vi "Z6_Beamline.color Beamline.vi"(0 "i ref in":refnum<vi>, 5 "error in (no error)":errorcluster) -> (14 "i ref out":refnum<vi>, 19 "error out":errorcluster)   [LabVIEW 2014, in "Z6_Beamline.lvlib"]
doc: "This VI sets the color of several beamline elements."
uses:
  Z6_Beamline.lvlib
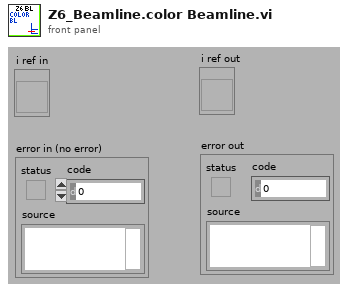
[diagram p1: front panel]
types:
  T1 = typedef "Z6_Beamline.lvlib/Z6_Beamline.i attribute.ctl" = cluster{"Subs ok GUI Refs":T2, "Refs BL Northtower":refnum<vi>[], "Refs BL Southtower":refnum<vi>[], "Refs BL 100TW COS":refnum<vi>[], "State Subsystems":cluster{"Northtower":bool, "Southtower":bool, "Frontends":bool, "100TW COS":bool}, "Z6 Beamline Status Subscriber Information":T3, "Color State PHELIX":i16}
  T2 = typedef "Z6_Beamline.lvlib/Z6_Beamline.Subsystem ok GUI Refs.ctl" = cluster{"Northtower ok":refnum<vi>, "Southtower ok":refnum<vi>, "Frontends ok":refnum<vi>, "100TW COS ok":refnum<vi>}
  T3 = typedef "Z6_Beamline.lvlib/Z6_Beamline.Status Subscriber Information.ctl" = cluster{"BL Z6 Shutter":T4, "CH 10":T4, "CH 11":T4, "ST Flip Cam":T4, "ST Flip DB":T4, "BL Z6 Dump":T4}
  T4 = typedef "PH_BL-Master.lvlib/PH_BL-Master.Status Subscriber Information.ctl" = cluster{"Index of element":i32, "Attributeset":T5}
  T5 = typedef "PH_BL-Master.lvlib/PH_BL-Master.Attribute Set.ctl" = enum16{"Boolean Status Service Subscriber", "Picture Status Service Subscriber"}
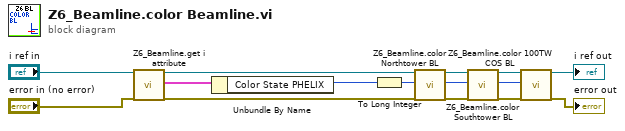
[diagram p0: block diagram]
diagram:
  n1 = call "Z6_Beamline.get i attribute.vi"("i ref in"="i ref in", "error in (no error)"="error in (no error)") -> ("i ref out"=w10:refnum<vi>, "i attribute"=w7:T1, "error out"=w8:errorcluster)  [unwired: 15 in]
  n2 = Unbundle By Name(w7) -> ("Color State PHELIX"=w6:i16)
  n3 = To Long Integer(number=w6) -> (32bit integer=w1:i32)
  n4 = call "Z6_Beamline.color Northtower BL.vi"("i ref in"=w10, "Color State Northtower Input"=w1, "error in (no error)"=w8) -> ("i ref out"=w15:refnum<vi>, "Color State Northwower Exit"=w12:i32, "error out"=w14:errorcluster)  [unwired: 14 in]
  n5 = call "Z6_Beamline.color Southtower BL.vi"("i ref in"=w15, "Color State Southtower Input"=w12, "error in (no error)"=w14) -> ("i ref out"=w4:refnum<vi>, "Color State Southwower Exit"=w2:i32, "error out"=w13:errorcluster)  [unwired: 14 in]
  n6 = call "Z6_Beamline.color 100TW COS BL.vi"("i ref in"=w4, "Color State 100TW COS Input"=w2, "error in (no error)"=w13) -> ("i ref out"=→"i ref out":refnum<vi>, "error out"=→"error out":errorcluster)  [unwired: 14 in, 1 out]
